vi "LV diagram wires.vi"(8 "error in (no error)":errorcluster, 11 "reference":refnum<vi>) -> (0 "error out":errorcluster, 3 "wiring":string)   [LabVIEW 2012]
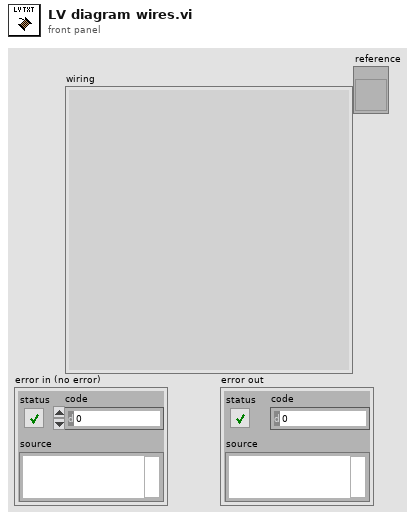
[diagram p1: front panel]
types:
  T1 = cluster{"UID":i32, "ClassID":u32, "ClassName":string, "Caption":string, "Name":string}
  T2 = cluster{"UID":i32, "ClassID":u32, "ClassName":string, "Desc":string, "Label.Text":string, cluster{"UID":i32, "ClassID":u32, "ClassName":string, "Caption":string, "Name":string}[]}
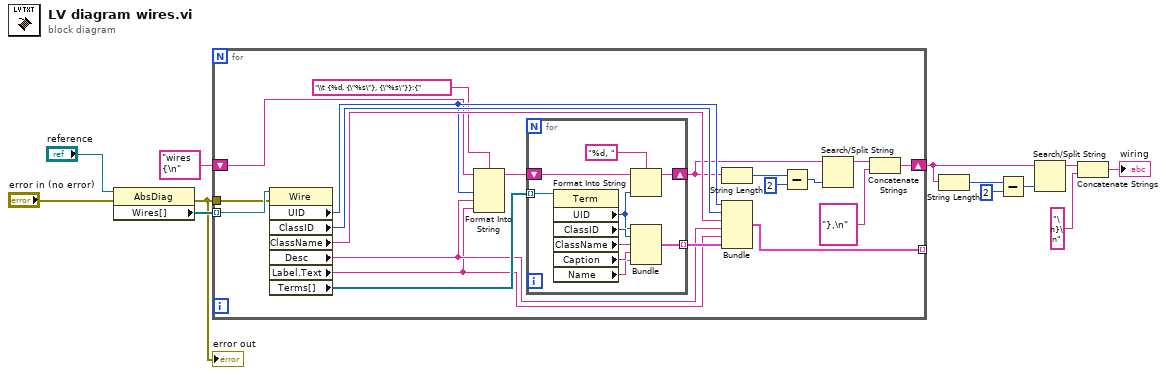
[diagram p0: block diagram]
diagram:
  n1 = property class="AbsDiag"(reference="reference", error in="error in (no error)") -> (error out=w11:errorcluster, "Wires[]"=w12:refnum<vi>[])  [unwired: 1 out]
  "error out" <- w11
  n2 = for {
    tunnel: w12 -> [w32] mode=indexing
    tunnel: [w29] -> _ mode=indexing
    tunnel: w11 -> [w26]
    shift-right: [w20] -> w4
    shift-left: "wires {\n" ("format string") -> [w24]
    n3 = property class="Wire"(reference=w32, error in=w26) -> ("UID"=w25:i32, "ClassID"=w31:u32, "ClassName"=w30:string, "Desc"=w14:string, "Label.Text"=w13:string, "Terms[]"=w28:refnum<vi>[])  [unwired: 2 out]
    n4 = Format Into String(format string="\\t {%d, {\"%s\"}, {\"%s\"}}:{", initial string=w24, w25, w14, w13) -> (resulting string=w22:string)  [unwired: 1 in, 1 out]
    n5 = for {
      tunnel: w28 -> [w42] mode=indexing
      tunnel: [w37] -> w27 mode=indexing
      shift-right: [w33] -> w19
      shift-left: w22 -> [w34]
      n6 = property class="Term"(reference=w42) -> ("UID"=w36:i32, "ClassID"=w41:u32, "ClassName"=w40:string, "Caption"=w39:string, "Name"=w38:string)  [unwired: 1 in, 2 out]
      n7 = Format Into String(format string="%d, ", initial string=w34, w36) -> (resulting string=w33:string)  [unwired: 1 in, 1 out]
      n8 = Bundle("UID"=w36, "ClassID"=w41, "ClassName"=w40, "Caption"=w39, "Name"=w38) -> (w37:T1)  [unwired: 1 in]
    }
    n9 = String Length(string=w19) -> (length=w18:i32)
    n10 = Bundle("UID"=w25, "ClassID"=w31, "ClassName"=w30, "Desc"=w14, "Label.Text"=w13, w27) -> (w29:T2)  [unwired: 1 in]
    n11 = Subtract(x=w18, y=2) -> (x-y=w16:i32)
    n12 = Search/Split String(string=w19, offset (0)=w16) -> (substring before match=w15:string)  [unwired: 1 in, 2 out]
    n13 = Concatenate Strings(w15, "},\n" ("format string")) -> (w20:string)
  }
  n14 = String Length(string=w4) -> (length=w5:i32)
  n15 = Subtract(x=w5, y=2) -> (x-y=w7:i32)
  n16 = Search/Split String(string=w4, offset (0)=w7) -> (substring before match=w3:string)  [unwired: 1 in, 2 out]
  n17 = Concatenate Strings(w3, "\n}\n" ("format string")) -> (→"wiring":string)
